vi "encoders to xy.vi"(9 "Red encoder":dbl, 10 "Blue encoder":dbl) -> (1 "X":dbl, 2 "Y":dbl)   [LabVIEW 2020]
panel:
  out "Red":dbl
  out "Red aa":dbl
  out "Blue angle":dbl
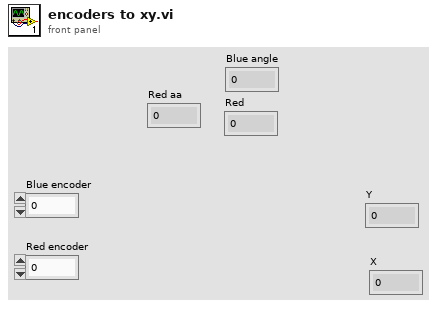
[diagram p1: front panel]
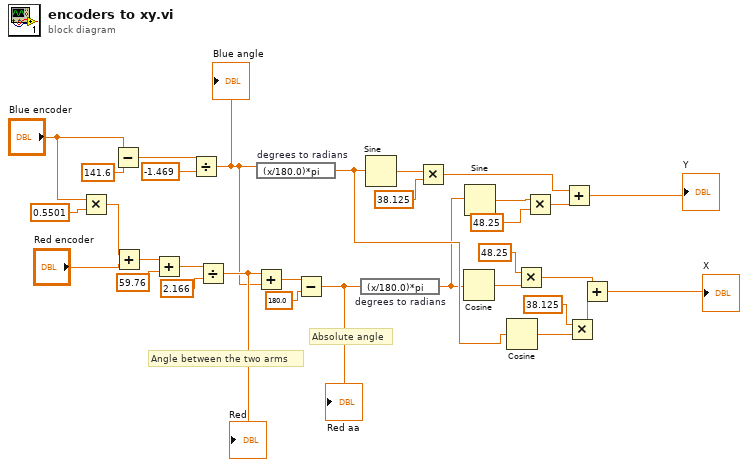
[diagram p0: block diagram]
diagram:
  # "Absolute angle"
  # "Angle between the two arms"
  n1 = Multiply(x="Blue encoder", y=0.5501) -> (x*y=w26:dbl)
  n2 = Subtract(x="Blue encoder", y=141.6) -> (x-y=w30:dbl)
  n3 = Add(x=w26, y="Red encoder") -> (x+y=w25:dbl)
  n4 = Add(x=w25, y=59.76) -> (x+y=w23:dbl)
  n5 = Divide(x=w30, y=-1.469) -> (x/y=w17:dbl)
  "Blue angle" <- w17
  n6 = Divide(x=w23, y=2.166) -> (x/y=w21:dbl)
  "Red" <- w21
  n7 = Add(x=w21, y=w17) -> (x+y=w20:dbl)
  n8 = expression code="(x/180.0)*pi" "degrees to radians"(w17) -> (w12:dbl)
  n9 = Subtract(x=w20, y=180.0) -> (x-y=w18:dbl)
  "Red aa" <- w18
  n10 = expression code="(x/180.0)*pi" "degrees to radians"(w18) -> (w7:dbl)
  n11 = Sine(x=w12) -> (sin(x)=w14:dbl)
  n12 = Multiply(x=w14, y=38.125) -> (x*y=w4:dbl)
  n13 = Cosine(x=w7) -> (cos(x)=w16:dbl)
  n14 = Sine(x=w7) -> (sin(x)=w5:dbl)
  n15 = Cosine(x=w12) -> (cos(x)=w10:dbl)
  n16 = Multiply(x=48.25, y=w16) -> (x*y=w9:dbl)
  n17 = Multiply(x=w5, y=48.25) -> (x*y=w3:dbl)
  n18 = Add(x=w4, y=w3) -> (x+y=→"Y":dbl)
  n19 = Multiply(x=38.125, y=w10) -> (x*y=w8:dbl)
  n20 = Add(x=w9, y=w8) -> (x+y=→"X":dbl)
